vi "UHR-Fleezers Control (host) - 12.0_test_fpga_connection.vi"() -> ()   [LabVIEW 2014] (continued)
                tunnel: w2776 -> [w2807]
                tunnel: w2785 -> [w2832]
                tunnel: w2786 -> [w2833]
                tunnel: w2780 -> [w2834]
                tunnel: w2777 -> [w2831]
                tunnel: [w2893] -> w2774
                frame #0 {
                  n1965 = local read "Trap Pos. FB ON"() -> (w2789:bool)
                  n1966 = Compound Arithmetic op=AND("Flow ON\nduring dip?", "FB OFF when \nflow ON", w2789) -> (w2790:bool)
                  n1967 = case shown="True" "Move trap \nbefore dip move?" {
                    frame False {
                    }
                    frame True {
                      n1968 = property on="Trap D (MHz)" class="DigNum (strict)"("Val(Sgnl)"="Dipping D (MHz)") -> ()  [unwired: 2 in, 2 out]
                    }
                  }
                  n1969 = property on="Green ON/Interlacing" class="Bool (strict)"("Val(Sgnl)"="Green ON\nbefore dip?") -> ()  [unwired: 2 in, 2 out]
                  n1970 = property on="Sample Channel\nFlow" class="Bool (strict)"("Val(Sgnl)"="Flow ON\nduring dip?") -> ()  [unwired: 2 in, 2 out]
                  n1971 = case shown="True" w2790 {
                    frame False {
                    }
                    frame True {
                      n1972 = property on="Trap Pos. FB ON" class="Bool (strict)"("Val(Sgnl)"=FALSE ("Value (Signaling)")) -> ()  [unwired: 2 in, 2 out]
                    }
                  }
                }
                frame #1 {
                  n1973 = local read "Saved Stage Positions"() -> (w2806:dbl[][])
                  n1974 = local write "Cancel dwell"(FALSE ("Cancel dwell")) -> ()
                  n1975 = call "move to saved stage position.vi"("error in"=w2804, "Stage VISA resource name in"=w2803, "Position"="Dip Stage \nPosition", "Saved Stage Positions"=w2806) -> ("VISA resource name out"=w2801:refnum<visa-resource-name>, "error out"=w2802:errorcluster)
                }
                frame #2 {
                  n1976 = node-c288() -> (w2810:T26)  [unwired: 4 in]
                  n1977 = timed-loop {
                    timing: w2810 -> [_]
                    timing-out: [_] -> w2809
                    tunnel: [w2816] -> w2808
                    i -> [w2813]
                    stop <- w2817 stop-if-true
                    n1978 = node-c288() -> ()  [unwired: 1 in, 1 out]
                    n1979 = Greater Or Equal?(x=w2813, y="Dip Duration (s)") -> (x >= y?=w2825:bool)
                    n1980 = local read "Dip for Protein"() -> (w2818:bool)
                    n1981 = local read "Dump Beads"() -> (w2815:bool)
                    n1982 = local read "Cancel dwell"() -> (w2824:bool)
                    n1983 = local read "Pause dwell"() -> (w2821:bool)
                    n1984 = Not(x=w2818) -> (.not. x?=w2823:bool)
                    n1985 = Compound Arithmetic op=OR(w2824, w2825, w2823) -> (w2822:bool)
                    n1986 = Select(t=FALSE, s=w2821, f=w2822) -> (s? t:f=w2819:bool)
                    n1987 = Not(x=w2815) -> (.not. x?=w2814:bool)
                    n1988 = node-c288() -> ()  [unwired: 1 in, 1 out]
                    n1989 = And(x=w2818, y=w2814) -> (x .and. y?=w2816:bool)
                    n1990 = Or(x=w2819, y=w2815) -> (x .or. y?=w2817:bool)
                    "Dip Time (s)" <- w2813
                  }
                  n1991 = node-c288(w2809) -> ()  [unwired: 1 out]
                }
                frame #3 {
                  n1992 = case shown="True" w2834 {
                    tunnel: w2833 -> [_ w2839]
                    tunnel: w2832 -> [_ w2838]
                    tunnel: w2831 -> [_ w2835]
                    frame False {
                    }
                    frame True {
                      n1993 = flat-sequence {
                        tunnel: w2838 -> [w2843]
                        tunnel: w2839 -> [w2844]
                        tunnel: [w2844] -> w2837
                        tunnel: [w2843] -> w2836
                        tunnel: w2835 -> [w2840]
                        tunnel: w2837 -> [w2854]
                        tunnel: w2836 -> [w2853]
                        tunnel: w2835 -> [w2862]
                        frame #0 {
                          n1994 = local read "Sample Channel\nFlow"() -> (w2842:bool)
                          n1995 = case shown="True" w2842 {
                            tunnel: "Flow ON \nduring return\nfrom dip?" -> [w2845 w2848]
                            tunnel: w2840 -> [_ w2847]
                            frame False {
                              n1996 = case shown="True" w2845 {
                                frame False {
                                }
                                frame True {
                                n1997 = property on="Sample Channel\nFlow" class="Bool (strict)"("Val(Sgnl)"=TRUE ("Value (Signaling)")) -> ()  [unwired: 2 in, 2 out]
                                }
                              }
                            }
                            frame True {
                              n1998 = case shown="False" w2848 {
                                tunnel: w2847 -> [w2849 _]
                                frame False {
                                n1999 = property on="Trap Pos. FB ON" class="Bool (strict)"("Val(Sgnl)"=w2849) -> ()  [unwired: 2 in, 2 out]
                                n2000 = property on="Sample Channel\nFlow" class="Bool (strict)"("Val(Sgnl)"=FALSE ("Value (Signaling)")) -> ()  [unwired: 2 in, 2 out]
                                }
                                frame True {
                                }
                              }
                            }
                          }
                        }
                        frame #1 {
                          # "For turning on green laser before stage reaches lower spot"
                          n2001 = case shown="True" "Green ON\nafter start\nreturn?" {
                            frame False {
                            }
                            frame True {
                              n2002 = flat-sequence {
                                frame #0 {
                                n2003 = Multiply(x="Green delay after \nstart return (s)", y=1000.0) -> (x*y=w2859:dbl)
                                n2004 = Wait (ms)(milliseconds to wait=w2859) -> ()  [unwired: 1 out]
                                }
                                frame #1 {
                                n2005 = property on="Green ON/Interlacing" class="Bool (strict)"("Val(Sgnl)"=TRUE ("Value (Signaling)")) -> ()  [unwired: 2 in, 2 out]
                                }
                              }
                            }
                          }
                          n2006 = local read "Saved Stage Positions"() -> (w2857:dbl[][])
                          n2007 = local write "Cancel dwell"(FALSE ("Cancel dwell")) -> ()
                          n2008 = call "move to saved stage position.vi"("error in"=w2853, "Stage VISA resource name in"=w2854, "Position"="Return Stage \nPosition", "Saved Stage Positions"=w2857) -> ("error out"=w2855:errorcluster)  [unwired: 1 out]
                          n2009 = local write "Stage Control Serial Error"(w2855) -> ()
                        }
                        frame #2 {
                          n2010 = property on="Trap Pos. FB ON" class="Bool (strict)"("Val(Sgnl)"=w2862) -> ()  [unwired: 2 in, 2 out]
                          n2011 = case shown="True" "Green ON \nafter return?" {
                            frame False {
                            }
                            frame True {
                              n2012 = property on="Green ON/Interlacing" class="Bool (strict)"("Val(Sgnl)"=TRUE ("Value (Signaling)")) -> ()  [unwired: 2 in, 2 out]
                            }
                          }
                          n2013 = case shown="True" "Move trap after return?" {
                            frame False {
                            }
                            frame True {
                              n2014 = property on="Trap D (MHz)" class="DigNum (strict)"("Val(Sgnl)"="Dip Trap D 2 (MHz)") -> ()  [unwired: 2 in, 2 out]
                            }
                          }
                          n2015 = case shown="True" "Save data after return?" {
                            frame False {
                            }
                            frame True {
                              n2016 = property on="Start Saving" class="Bool (strict)"("Val(Sgnl)"=TRUE ("Value (Signaling)")) -> ()  [unwired: 2 in, 2 out]
                            }
                          }
                          n2017 = property on="Sample Channel\nFlow" class="Bool (strict)"("Val(Sgnl)"="Flow ON\nduring daq?") -> ()  [unwired: 2 in, 2 out]
                        }
                        frame #3 {
                          n2018 = node-c288() -> (w2871:T26)  [unwired: 4 in]
                          n2019 = timed-loop {
                            timing: w2871 -> [_]
                            timing-out: [_] -> w2870
                            i -> [w2872]
                            stop <- w2874 stop-if-true
                            n2020 = node-c288() -> ()  [unwired: 1 in, 1 out]
                            n2021 = local read "Dump Beads"() -> (w2873:bool)
                            n2022 = Greater Or Equal?(x=w2872, y="Dwell Duration (s)") -> (x >= y?=w2879:bool)
                            n2023 = local read "Dip for Protein"() -> (w2876:bool)
                            n2024 = Not(x=w2876) -> (.not. x?=w2875:bool)
                            n2025 = Compound Arithmetic op=OR(w2879, "Cancel dwell", w2875) -> (w2878:bool)
                            n2026 = node-c288() -> ()  [unwired: 1 in, 1 out]
                            n2027 = Select(t=FALSE, s="Pause dwell", f=w2878) -> (s? t:f=w2881:bool)
                            n2028 = Or(x=w2881, y=w2873) -> (x .or. y?=w2874:bool)
                            "Dwell Time (s)" <- w2872
                          }
                          n2029 = node-c288(w2870) -> ()  [unwired: 1 out]
                        }
                      }
                    }
                  }
                }
                frame #4 {
                  n2030 = local read "Dip for Protein"() -> (w2890:bool)
                  n2031 = local read "Tether"() -> (w2889:bool)
                  n2032 = local read "Dump Beads"() -> (w2891:bool)
                  n2033 = local write "Cancel dwell"(FALSE ("Cancel dwell")) -> ()
                  n2034 = Not(x=w2889) -> (.not. x?=w2888:bool)
                  n2035 = Not(x=w2890) -> (.not. x?=w2894:bool)
                  n2036 = Not(x="Cont. Repeat Dipping?") -> (.not. x?=w2896:bool)
                  n2037 = Compound Arithmetic op=OR(w2888, w2894, w2896, w2891) -> (w2893:bool)
                }
              }
            }
          }
        }
      }
      event "Profile": Value Change {
        n2038 = event-data() -> ()  [unwired: 1 in, 5 out]
        n2039 = flat-sequence {
          tunnel: w2905 -> [w2908]
          tunnel: w2904 -> [w2916]
          tunnel: [w2910] -> w2903
          tunnel: [w2909] -> w2902
          tunnel: [w2907] -> w2900
          tunnel: [w2906] -> w2897
          tunnel: w2903 -> [w2923]
          tunnel: w2902 -> [w2922]
          tunnel: [w2920] -> w2901
          tunnel: w2900 -> [w2921]
          tunnel: [w2919] -> w2899
          tunnel: [w2918] -> w2898
          tunnel: w2897 -> [w2918]
          tunnel: w2901 -> [w2927]
          tunnel: w2899 -> [w2926]
          tunnel: w2898 -> [w2925]
          frame #0 {
            n2040 = call "Read Stage Position.vi"("error in"=w2916, "VISA resource name in"=w2908) -> ("Current Position"=w2906:cluster{dbl, dbl, dbl}, "error out"=w2909:errorcluster, "VISA resource name out"=w2907:refnum<visa-resource-name>)  [unwired: 1 out]
            "Current Position" <- w2906
            n2041 = local write "Stage Control Serial Error"(w2909) -> ()
            n2042 = Unbundle(w2906) -> (w2913:dbl, w2915:dbl, w2911:dbl)
            n2043 = Add(x=w2915, y="Y change (mm)") -> (x+y=w2912:dbl)
            n2044 = Bundle(w2913, w2912, w2911) -> (w2910:cluster{dbl, dbl, dbl})  [unwired: 1 in]
          }
          frame #1 {
            # "move to new position and start saving"
            n2045 = local write "Stage Moving"(TRUE ("Stage Moving")) -> ()
            n2046 = local write "Start Saving"(TRUE ("Start Saving")) -> ()
            n2047 = call "Set Stage Position.vi"("Position"=w2923, "error in"=w2922, "VISA resource name in"=w2921) -> ("error out"=w2919:errorcluster, "VISA resource name out"=w2920:refnum<visa-resource-name>)  [unwired: 1 out]
          }
          frame #2 {
            # "go back to start"
            n2048 = call "Set Stage Position.vi"("Position"=w2925, "error in"=w2926, "VISA resource name in"=w2927) -> ()  [unwired: 3 out]
          }
          frame #3 {
            # "stop saving"
            n2049 = local write "Stop Saving"(TRUE ("Stop Saving")) -> ()
            n2050 = local write "Stage Moving"(FALSE ("Stage Moving")) -> ()
          }
        }
      }
      event "Move to Position 1", "Move to Position 2", "Move to Position 3", "Move to Position 4", "Move to Position 5", "Lower Ch. Cap.": Value Change {
        n2051 = event-data() -> ()  [unwired: 1 in, 5 out]
        n2052 = Or(x="Move to Position 5", y="Lower Ch. Cap.") -> (x .or. y?=w2933:bool)
        n2053 = Build Array("Move to Position 1", "Move to Position 2", "Move to Position 3", "Move to Position 4", w2933) -> (w2936:bool[])
        n2054 = Boolean Array To Number(Boolean array=w2936) -> (number=w2935:u32)
        n2055 = Logarithm Base 2(1:w2935) -> (0:w2934:dbl)
        n2056 = flat-sequence {
          tunnel: w2934 -> [w2945]
          tunnel: w2931 -> [w2943]
          tunnel: w2930 -> [w2942]
          frame #0 {
            n2057 = local read "Saved Stage Positions"() -> (w2953:dbl[][])
            n2058 = Array Subset(array=w2953, index (row)=w2945, length (row)=1 ("length"), index (col)=1 ("index"), length (col)=3 ("length")) -> (w2950:dbl[][])
            n2059 = Reshape Array(w2950, 3 ("dimension size")) -> (w2948:dbl[])
            n2060 = Array To Cluster(array=w2948) -> (cluster=w2947:cluster{"[0]":dbl, "[1]":dbl, "[2]":dbl})
            n2061 = call "Set Stage Position.vi"("Position"=w2947, "error in"=w2942, "VISA resource name in"=w2943) -> ("error out"=w2946:errorcluster)  [unwired: 2 out]
            n2062 = local write "Stage Moving"(TRUE ("Stage Moving")) -> ()
            n2063 = local write "Stage Control Serial Error"(w2946) -> ()
          }
          frame #1 {
            n2064 = local write "Stage Moving"(FALSE ("Stage Moving")) -> ()
            n2065 = call <vilib>:"Beep.vi"() -> ()  [unwired: 3 in, 9 out]
          }
        }
      }
      event "Set Current\nPos to 0,0,0": Value Change {
        # "DH is \"Define Home\""
        n2066 = event-data() -> ()  [unwired: 1 in, 6 out]
        n2067 = local write "Set Current\nPos to 0,0,0"(FALSE ("Set Current\nPos to 0,0,0")) -> ()
        n2068 = Concatenate Strings("1DH" ("string"), ";" ("string"), "2DH" ("string"), ";" ("string"), "3DH" ("string"), "\r") -> (w2961:string)
        n2069 = call-poly "VISA Configure Serial Port"("VISA resource name"=w2966, "baud rate (9600)"=u32 19200, "error in (no error)"=w2965) -> ("VISA resource name out"=w2963:refnum<visa-resource-name>, "error out"=w2962:errorcluster)  [unwired: 11 in]
        n2070 = VISA Write(VISA resource name=w2963, write buffer=w2961, error in (no error)=w2962) -> (error out=w2956:errorcluster)  [unwired: 2 out]
        n2071 = local write "Stage Control Serial Error"(w2956) -> ()
      }
      event "Got ADig bead": Value Change {
        n2072 = event-data() -> ()  [unwired: 1 in, 5 out]
        n2073 = flat-sequence {
          frame #0 {
            n2074 = local read "Cap 1 Samp Flow ON"() -> (w2972:bool)
            n2075 = case shown="True" w2972 {
              frame False {
              }
              frame True {
                n2076 = property on="Sample Channel\nFlow" class="Bool (strict)"("Val(Sgnl)"=TRUE ("Value (Signaling)")) -> ()  [unwired: 2 in, 2 out]
              }
            }
            n2077 = local write "Got ADig bead"(FALSE) -> ()
          }
          frame #1 {
            n2078 = property on="Inject Pump 3" class="Bool (strict)"("Val(Sgnl)"=FALSE ("Value (Signaling)")) -> ()  [unwired: 2 in, 2 out]
            n2079 = local write "Target"(FALSE ("Target")) -> ()
          }
          frame #2 {
            n2080 = property on="Move Cap. 1 (DNA Bottom)" class="Bool (strict)"("Val(Sgnl)"=TRUE ("Value (Signaling)")) -> ()  [unwired: 2 in, 2 out]
          }
        }
      }
      event "Force FB Script": Value Change {
        n2081 = event-data() -> ()  [unwired: 1 in, 5 out]
        n2082 = local write "Force FB Script"(FALSE ("Force FB Data\nScript")) -> ()
        n2083 = flat-sequence {
          tunnel: w2983 -> [w2987]
          tunnel: w2984 -> [w2988]
          tunnel: [w2988] -> w2979
          tunnel: [w2987] -> w2978
          tunnel: w2979 -> [w2991]
          tunnel: w2978 -> [w2990]
          tunnel: ["Trap Trig Fl."] -> w2980
          tunnel: [w3033] -> w2981
          tunnel: w2980 -> [w3033]
          tunnel: [w3037] -> w2982
          tunnel: w2981 -> [w3037]
          tunnel: w2982 -> [w3039]
          frame #0 {
            n2084 = property on="Trap D (MHz)" class="DigNum (strict)"("Val(Sgnl)"="Trap D Before Moving") -> ()  [unwired: 2 in, 2 out]
          }
          frame #1 {
            n2085 = local read "Saved Stage Positions"() -> (w2993:dbl[][])
            n2086 = local write "FB Trap Pos Offset"(0.0 ("FB Trap Pos Offset")) -> ()
            n2087 = property on="Trap Pos. FB Offset Factor" class="DigNum (strict)"("Val(Sgnl)"=i64 0 ("Value (Signaling)")) -> ()  [unwired: 2 in, 2 out]
            n2088 = local write "Stage Moving"(TRUE ("Stage Moving")) -> ()
            n2089 = call "move to saved stage position.vi"("error in"=w2990, "Stage VISA resource name in"=w2991, "Position"="Stage Position To Establish FB", "Saved Stage Positions"=w2993) -> ("error out"=w2989:errorcluster)  [unwired: 1 out]
            n2090 = local write "Stage Control Serial Error"(w2989) -> ()
          }
          frame #2 {
            n2091 = call <vilib>:"Beep.vi"("duration (msec)"=u32 100, "frequency (Hz)"=u32 20) -> ()  [unwired: 1 in, 9 out]
            n2092 = local write "Stage Moving"(FALSE ("Stage Moving")) -> ()
            n2093 = property on="Tab Control 2" class="TabCtl (strict)"("Val(Sgnl)"=T6."Feedback on Trap Position" ("Value (Signaling)")) -> ()  [unwired: 2 in, 2 out]
            n2094 = stacked-sequence {
              frame #0 {
                n2095 = Multiply(x="Wait (s)", y=u32 1000 ("milliseconds to wait")) -> (x*y=w3002:u32)
                n2096 = property on="Trap D (MHz)" class="DigNum (strict)"("Val(Sgnl)"="Starting Trap D (MHz)") -> ()  [unwired: 2 in, 2 out]
                n2097 = Wait (ms)(milliseconds to wait=w3002) -> ()  [unwired: 1 out]
              }
              frame #1 {
                n2098 = property on="Set Reading to\nSetpoint" class="Bool (strict)"("Val(Sgnl)"=TRUE ("Value (Signaling)")) -> ()  [unwired: 2 in, 2 out]
              }
            }
            n2099 = property on="Tab Control" class="TabCtl (strict)"("Val(Sgnl)"=T34."Trap Control (RF)" ("Value (Signaling)")) -> ()  [unwired: 2 in, 2 out]
          }
          frame #3 {
            n2100 = Wait (ms)(milliseconds to wait=u32 500) -> ()  [unwired: 1 out]
          }
          frame #4 {
            n2101 = property on="Trap Pos. FB ON" class="Bool (strict)"("Val(Sgnl)"=TRUE ("Value (Signaling)")) -> ()  [unwired: 2 in, 2 out]
            n2102 = Wait (ms)(milliseconds to wait=u32 250) -> ()  [unwired: 1 out]
          }
          frame #5 {
            n2103 = case shown="\"1\"" "Remove Action Offset Dropdown" {
              tunnel: TRUE ("Value (Signaling)") -> [w3014 w3022 w3030]
              frame "1" {
                n2104 = flat-sequence {
                  tunnel: w3014 -> [w3021]
                  frame #0 {
                    n2105 = local read "factor"() -> (w3016:dbl)
                    n2106 = Greater Than 0?(x=w3016) -> (x > 0?=w3020:bool)
                    n2107 = Select(t=1.0, s=w3020, f=-1.0) -> (s? t:f=w3017:dbl)
                    n2108 = Multiply(x=w3017, y=w3016) -> (x*y=w3015:dbl)
                    n2109 = local write "factor"(w3015) -> ()
                  }
                  frame #1 {
                    n2110 = property on="Remove Offset to factor" class="Bool (strict)"("Val(Sgnl)"=w3021) -> ()  [unwired: 2 in, 2 out]
                  }
                }
              }
              frame "2" {
                n2111 = flat-sequence {
                  tunnel: w3022 -> [w3029]
                  frame #0 {
                    n2112 = local read "factor"() -> (w3023:dbl)
                    n2113 = Greater Than 0?(x=w3023) -> (x > 0?=w3028:bool)
                    n2114 = Select(t=-1.0, s=w3028, f=1.0) -> (s? t:f=w3026:dbl)
                    n2115 = Multiply(x=w3023, y=w3026) -> (x*y=w3025:dbl)
                    n2116 = local write "factor"(w3025) -> ()
                  }
                  frame #1 {
                    n2117 = property on="Remove Offset to factor" class="Bool (strict)"("Val(Sgnl)"=w3029) -> ()  [unwired: 2 in, 2 out]
                  }
                }
              }
              frame "0", Default {
                n2118 = property on="Remove Action Offset" class="Bool (strict)"("Val(Sgnl)"=w3030) -> ()  [unwired: 2 in, 2 out]
              }
            }
            n2119 = case shown="False" "Trap Trig Fl." {
              frame False {
                n2120 = case shown="True" "Green ON after FB ON?" {
                  selector: "Green ON after FB ON?" -> [_ w3032]
                  frame False {
                  }
                  frame True {
                    n2121 = property on="Green ON/Interlacing" class="Bool (strict)"("Val(Sgnl)"=w3032) -> ()  [unwired: 2 in, 2 out]
                  }
                }
              }
              frame True {
              }
            }
            n2122 = Wait (ms)(milliseconds to wait=u32 250) -> ()  [unwired: 1 out]
          }
          frame #6 {
            n2123 = property on="Start Saving" class="Bool (strict)"("Val(Sgnl)"=TRUE ("Value (Signaling)")) -> ()  [unwired: 2 in, 2 out]
            n2124 = Wait (ms)(milliseconds to wait=u32 5000) -> ()  [unwired: 1 out]
          }
          frame #7 {
            w3036 = TRUE ("Value (Signaling)")
            n2125 = property on="Rem fb disp offset" class="Bool (strict)"("Val(Sgnl)"=w3036) -> ()  [unwired: 2 in, 2 out]
            n2126 = property on="Remove Offset" class="Bool (strict)"("Val(Sgnl)"=w3036) -> ()  [unwired: 2 in, 2 out]
            n2127 = Wait (ms)(milliseconds to wait=u32 100) -> ()  [unwired: 1 out]
          }
          frame #8 {
            n2128 = case shown="True" w3039 {
              frame False {
              }
              frame True {
                n2129 = local write "Trap Trig. Fl."(TRUE ("Value (Signaling)")) -> ()
              }
            }
          }
          frame #9 {
            n2130 = local read "Tether"() -> (w3042:bool)
            n2131 = And(x="Start dipping after?", y=w3042) -> (x .and. y?=w3041:bool)
            n2132 = case shown="True" w3041 {
              frame False {
              }
              frame True {
                n2133 = flat-sequence {
                  frame #0 {
                    n2134 = Multiply(x="Delay before dipping (s)", y=1000.0) -> (x*y=w3045:dbl)
                    n2135 = Wait (ms)(milliseconds to wait=w3045) -> ()  [unwired: 1 out]
                  }
                  frame #1 {
                    n2136 = property on="Dip for Protein" class="Bool (strict)"("Val(Sgnl)"=TRUE ("Value (Signaling)")) -> ()  [unwired: 2 in, 2 out]
                    n2137 = local write "Scripts"(T35."Dipping") -> ()
                  }
                }
              }
            }
          }
        }
      }
      event "Rupture Script": Value Change {
        n2138 = event-data() -> ()  [unwired: 1 in, 5 out]
        n2139 = local write "Rupture Script"(FALSE ("Rupture Script")) -> ()
        n2140 = flat-sequence {
          frame #0 {
            w3051 = TRUE
            w3056 = FALSE
            # "Number 6 for now is the\nrupture-experiment\nparameters."
            n2141 = local read "Starting Trap D (MHz)"() -> (w3057:dbl)
            n2142 = local write "Restart DMA? (AOD)"(w3056) -> ()
            n2143 = Replace Array Subset(array=u32[] [0] ("Index Values"), new element=6, index=0) -> (w3052:u32[])
            n2144 = local write "Save scans"(w3056) -> ()
            n2145 = property on="Trap D (MHz)" class="DigNum (strict)"("Val(Sgnl)"=w3057) -> ()  [unwired: 2 in, 2 out]
            n2146 = property on="Saved AOD Raster Scan Parameter Sets" class="Arr (strict)"("Index Values"=w3052) -> ()  [unwired: 2 in, 2 out]
            n2147 = property on="Start Saving" class="Bool (strict)"("Val(Sgnl)"=w3051) -> ()  [unwired: 2 in, 2 out]
            n2148 = property on="Green ON/Interlacing" class="Bool (strict)"("Val(Sgnl)"=w3051) -> ()  [unwired: 2 in, 2 out]
          }
          frame #1 {
            n2149 = property on="Load parameters" class="Bool (strict)"("Val(Sgnl)"=TRUE ("Value (Signaling)")) -> ()  [unwired: 2 in, 2 out]
          }
        }
      }
      event "Fixed Traps Script": Value Change {
        n2150 = event-data() -> ()  [unwired: 1 in, 5 out]
        n2151 = local write "Fixed Traps Script"(FALSE ("Fixed Traps Data\nScript")) -> ()
        n2152 = flat-sequence {
          frame #0 {
            n2153 = case shown="True" "Green ON" {
              frame False {
              }
              frame True {
                n2154 = property on="Green ON/Interlacing" class="Bool (strict)"("Val(Sgnl)"=TRUE) -> ()  [unwired: 2 in, 2 out]
              }
            }
            n2155 = local write "Offset (nm)"(0.0 ("Offset (nm)")) -> ()
            n2156 = property on="Sample Channel\nFlow" class="Bool (strict)"("Val(Sgnl)"=FALSE ("Value (Signaling)")) -> ()  [unwired: 2 in, 2 out]
            n2157 = property on="Trap D (MHz)" class="DigNum (strict)"("Val(Sgnl)"="Fixed Traps Trap Delta (MHz)") -> ()  [unwired: 2 in, 2 out]
          }
          frame #1 {
            n2158 = Wait (ms)(milliseconds to wait=u32 1000) -> ()  [unwired: 1 out]
          }
          frame #2 {
            n2159 = local write "Start Saving"(TRUE ("Start Saving")) -> ()
          }
          frame #3 {
            n2160 = local read "Bead Sep. Int. Time (s)"() -> (w3067:dbl)
            n2161 = Multiply(x=w3067, y=1000.0) -> (x*y=w3069:dbl)
            n2162 = Wait (ms)(milliseconds to wait=w3069) -> ()  [unwired: 1 out]
          }
          frame #4 {
            n2163 = property on="Remove Offset" class="Bool (strict)"("Val(Sgnl)"=TRUE ("Value (Signaling)")) -> ()  [unwired: 2 in, 2 out]
          }
          frame #5 {
            n2164 = property on="Dip for Protein" class="Bool (strict)"("Val(Sgnl)"="Start dipping after?") -> ()  [unwired: 2 in, 2 out]
          }
        }
      }
      event "Got DNA bead": Value Change {
        n2165 = event-data() -> ()  [unwired: 1 in, 5 out]
        n2166 = flat-sequence {
          frame #0 {
            w3073 = FALSE ("Key Focus")
            n2167 = local read "Daq spot flow on"() -> (w3074:bool)
            n2168 = case shown="True" w3074 {
              frame False {
              }
              frame True {
                n2169 = property on="Sample Channel\nFlow" class="Bool (strict)"("Val(Sgnl)"=TRUE ("Value (Signaling)")) -> ()  [unwired: 2 in, 2 out]
              }
            }
            n2170 = local write "Got DNA bead"(w3073) -> ()
            n2171 = property on="Got DNA bead" class="Bool (strict)"("Key Focus"=w3073) -> ()  [unwired: 2 in, 2 out]
          }
          frame #1 {
            n2172 = property on="Inject Pump 1" class="Bool (strict)"("Val(Sgnl)"=FALSE ("Value (Signaling)")) -> ()  [unwired: 2 in, 2 out]
          }
          frame #2 {
            n2173 = property on="Cal/Data Acq. Spot" class="Bool (strict)"("Val(Sgnl)"=TRUE ("Value (Signaling)")) -> ()  [unwired: 2 in, 2 out]
          }
        }
      }
      event "Take Stepping Data": Value Change {
        n2174 = event-data() -> ()  [unwired: 1 in, 5 out]
        n2175 = local read "Save ave N"() -> (w3086:dbl)
        n2176 = flat-sequence {
          tunnel: w3086 -> [w3088]
          tunnel: [w3088] -> w3081
          tunnel: [w3090] -> w3082
          tunnel: w3081 -> [w3090]
          tunnel: [w3092] -> w3083
          tunnel: w3082 -> [w3092]
          tunnel: [w3095] -> w3084
          tunnel: w3083 -> [w3095]
          tunnel: [w3097] -> w3085
          tunnel: w3084 -> [w3097]
          tunnel: [w3099] -> w3079
          tunnel: w3085 -> [w3099]
          tunnel: w3079 -> [w3102]
          tunnel: [w3102] -> w3078
          tunnel: w3078 -> [w3103]
          tunnel: [w3103] -> w3080
          tunnel: w3080 -> [w3109]
          frame #0 {
            n2177 = property on="Save ave N" class="DigNum (strict)"("Val(Sgnl)"="Save ave factor") -> ()  [unwired: 2 in, 2 out]
          }
          frame #1 {
            n2178 = Wait (ms)(milliseconds to wait=u32 100) -> ()  [unwired: 1 out]
          }
          frame #2 {
            n2179 = local read "Offset 2 Start (MHz)"() -> (w3094:dbl)
            n2180 = property on="Saved AOD Raster Scan Parameter Sets" class="Arr (strict)"("Index Values"=u32[] [2]) -> ()  [unwired: 2 in, 2 out]
            n2181 = property on="Trap D (MHz)" class="DigNum (strict)"("Val(Sgnl)"=w3094) -> ()  [unwired: 2 in, 2 out]
          }
          frame #3 {
            n2182 = property on="Load parameters" class="Bool (strict)"("Val(Sgnl)"=TRUE ("Value (Signaling)")) -> ()  [unwired: 2 in, 2 out]
          }
          frame #4 {
            n2183 = Wait (ms)(milliseconds to wait=u32 100) -> ()  [unwired: 1 out]
          }
          frame #5 {
            n2184 = property on="Trap Raster Scan" class="Bool (strict)"("Val(Sgnl)"=TRUE ("Value (Signaling)")) -> ()  [unwired: 2 in, 2 out]
          }
          frame #6 {
            n2185 = Wait (ms)(milliseconds to wait=u32 1000) -> ()  [unwired: 1 out]
          }
          frame #7 {
            n2186 = while {
              stop <- w3106 stop-if-true
              n2187 = local read "Raster Scanning..."() -> (w3108:bool)
              n2188 = local read "Saving..."() -> (w3107:bool)
              n2189 = Not(x=w3107) -> (.not. x?=w3104:bool)
              n2190 = Not(x=w3108) -> (.not. x?=w3105:bool)
              n2191 = And(x=w3105, y=w3104) -> (x .and. y?=w3106:bool)
            }
          }
          frame #8 {
            n2192 = property on="Save ave N" class="DigNum (strict)"("Val(Sgnl)"=w3109) -> ()  [unwired: 2 in, 2 out]
          }
        }
      }
      event "Step Size (nm)": Value Change {
        n2193 = event-data() -> ()  [unwired: 1 in, 5 out]
        n2194 = flat-sequence {
          frame #0 {
            n2195 = property on="Saved AOD Raster Scan Parameter Sets" class="Arr (strict)"("Index Values"=u32[] [1]) -> ()  [unwired: 2 in, 2 out]
          }
          frame #1 {
            n2196 = Multiply(x="N Steps", y="Step Size (nm)") -> (x*y=w3111:dbl)
            n2197 = property on="Scan Speed AOD (nm/s) 2" class="DigNum (strict)"("Value"="Step Size (nm)") -> ()  [unwired: 2 in, 2 out]
            n2198 = property on="Step Size AOD (nm) 2" class="DigNum (strict)"("Value"="Step Size (nm)") -> ()  [unwired: 2 in, 2 out]
            n2199 = property on="Scan Range AOD (nm) 2" class="DigNum (strict)"("Value"=w3111) -> ()  [unwired: 2 in, 2 out]
          }
        }
      }
      event "Take Detection Laser\nImage": Value Change {
        n2200 = event-data() -> ()  [unwired: 1 in, 5 out]
        n2201 = flat-sequence {
          tunnel: [w3139] -> w3129
          tunnel: [w3138] -> w3122
          tunnel: [w3137] -> w3114
          tunnel: [w3142] -> w3130
          tunnel: w3129 -> [w3142]
          tunnel: [w3141] -> w3123
          tunnel: w3122 -> [w3141]
          tunnel: [w3140] -> w3115
          tunnel: w3114 -> [w3140]
          tunnel: [w3146] -> w3131
          tunnel: w3130 -> [w3146]
          tunnel: [w3145] -> w3124
          tunnel: w3123 -> [w3145]
          tunnel: [w3144] -> w3116
          tunnel: w3115 -> [w3144]
          tunnel: [w3152] -> w3132
          tunnel: w3131 -> [w3152]
          tunnel: [w3151] -> w3125
          tunnel: w3124 -> [w3151]
          tunnel: [w3150] -> w3117
          tunnel: w3116 -> [w3150]
          tunnel: [w3156] -> w3133
          tunnel: w3132 -> [w3156]
          tunnel: [w3155] -> w3126
          tunnel: w3125 -> [w3155]
          tunnel: [w3154] -> w3118
          tunnel: w3117 -> [w3154]
          tunnel: [w3160] -> w3134
          tunnel: w3133 -> [w3160]
          tunnel: [w3159] -> w3127
          tunnel: w3126 -> [w3159]
          tunnel: [w3158] -> w3119
          tunnel: w3118 -> [w3158]
          tunnel: [w3164] -> w3135
          tunnel: w3134 -> [w3164]
          tunnel: [w3163] -> w3128
          tunnel: w3127 -> [w3163]
          tunnel: [w3162] -> w3120
          tunnel: w3119 -> [w3162]
          tunnel: w3135 -> [w3170]
          tunnel: w3128 -> [w3169]
          tunnel: [w3167] -> w3121
          tunnel: w3120 -> [w3167]
          tunnel: w3121 -> [w3171]
          frame #0 {
            n2202 = local read "Laser interlacing mode (all lasers)"() -> (w3138:enum32{"Laser ON", "Laser OFF", "Interlace"})
            n2203 = local read "Green ON/Interlacing"() -> (w3139:bool)
            n2204 = local read "Green FB On/Off"() -> (w3137:bool)
          }
          frame #1 {
            n2205 = property on="Green FB On/Off" class="Bool (strict)"("Val(Sgnl)"=FALSE ("Value (Signaling)")) -> ()  [unwired: 2 in, 2 out]
          }
          frame #2 {
            n2206 = property on="Green ON/Interlacing" class="Bool (strict)"("Val(Sgnl)"=TRUE ("Value (Signaling)")) -> ()  [unwired: 2 in, 2 out]
            n2207 = property on="Flip Green Filter" class="Bool (strict)"("Val(Sgnl)"=TRUE ("Value (Signaling)")) -> ()  [unwired: 2 in, 2 out]
            n2208 = property on="Laser interlacing mode (all lasers)" class="RadioBtnsControl (strict)"("Val(Sgnl)"=enum32{"Laser ON", "Laser OFF", "Interlace"}."Laser ON" ("Value (Signaling)")) -> ()  [unwired: 2 in, 2 out]
          }
          frame #3 {
            n2209 = Wait (ms)(milliseconds to wait=u32 500) -> ()  [unwired: 1 out]
          }
          frame #4 {
            n2210 = property on="Confocal\nImage" class="Bool (strict)"("Val(Sgnl)"=TRUE ("Value (Signaling)")) -> ()  [unwired: 2 in, 2 out]
          }
          frame #5 {
            n2211 = Wait (ms)(milliseconds to wait=u32 2000) -> ()  [unwired: 1 out]
          }
          frame #6 {
            n2212 = while {
              stop <- w3165 stop-if-true
              n2213 = local read "Saving..."() -> (w3166:bool)
              n2214 = Not(x=w3166) -> (.not. x?=w3165:bool)
            }
          }
          frame #7 {
            n2215 = property on="Flip Green Filter" class="Bool (strict)"("Val(Sgnl)"=TRUE ("Value (Signaling)")) -> ()  [unwired: 2 in, 2 out]
            n2216 = property on="Green ON/Interlacing" class="Bool (strict)"("Val(Sgnl)"=w3170) -> ()  [unwired: 2 in, 2 out]
            n2217 = property on="Laser interlacing mode (all lasers)" class="RadioBtnsControl (strict)"("Val(Sgnl)"=w3169) -> ()  [unwired: 2 in, 2 out]
          }
          frame #8 {
            n2218 = property on="Green FB On/Off" class="Bool (strict)"("Val(Sgnl)"=w3171) -> ()  [unwired: 2 in, 2 out]
          }
        }
      }
      event "Stop All": Value Change {
        n2219 = event-data() -> ()  [unwired: 1 in, 5 out]
        n2220 = local read "Stop All"() -> (w3172:bool)
      }
    }
    n2221 = node-c288() -> ()  [unwired: 1 in, 1 out]
  }
  n2222 = node-c288() -> (w139:T26)  [unwired: 4 out]
  n2223 = timed-loop "Mouse control: trap position (AOM deflection), set confocal spot from image" {
    tunnel: [w3174] -> w224
    tunnel: w51 -> [w3173]
    timing: w139 -> [_]
    timing-out: [_] -> w138
    stop <- w3174 stop-if-true
    n2224 = node-c288() -> ()  [unwired: 2 out]
    n2225 = event shown="[0] \"Pane\": Mouse Down" {
      selector: _ -> [_ _]
      dyn-events: _ -> [_ _]
      timeout: _ -> [_ _]
      tunnel: w3173 -> [w3177 _]
      event Mouse Down {
        n2226 = event-data() -> ("Time"=w3179:u32, "Coords"=w3178:T7, "Button"=w3180:u16)  [unwired: 6 out]
        n2227 = case shown="1" w3180 {
          tunnel: w3179 -> [_ _ w3319]
          tunnel: w3178 -> [_ w3185 w3317]
          tunnel: w3177 -> [_ _ w3315]
          frame 0, Default {
          }
          frame 1 {
            n2228 = property on="APD 2" class="ImageControl"() -> ("Displayed Image Position"=w3199:cluster{"Left":i32, "Top":i32})  [unwired: 2 in, 2 out]
            n2229 = control-ref of="Primary Video Display"() -> (w3192:refnum<vi>)
            n2230 = property on="APD 1" class="ImageControl"() -> ("Displayed Image Position"=w3228:cluster{"Left":i32, "Top":i32})  [unwired: 2 in, 2 out]
            n2231 = property on="Detection Laser X" class="ImageControl"() -> ("Displayed Image Position"=w3225:cluster{"Left":i32, "Top":i32})  [unwired: 2 in, 2 out]
            n2232 = property on="Detection Laser Y" class="ImageControl"() -> ("Displayed Image Position"=w3224:cluster{"Left":i32, "Top":i32})  [unwired: 2 in, 2 out]
            n2233 = property on="APD 2" class="ImageControl"() -> ("Displayed Image Size"=w3198:cluster{"Width":u32, "Height":u32})  [unwired: 2 in, 2 out]
            n2234 = property on="APD 1" class="ImageControl"() -> ("Displayed Image Size"=w3226:cluster{"Width":u32, "Height":u32})  [unwired: 2 in, 2 out]
            n2235 = property on="Detection Laser X" class="ImageControl"() -> ("Displayed Image Size"=w3227:cluster{"Width":u32, "Height":u32})  [unwired: 2 in, 2 out]
            n2236 = property on="Detection Laser Y" class="ImageControl"() -> ("Displayed Image Size"=w3223:cluster{"Width":u32, "Height":u32})  [unwired: 2 in, 2 out]
            n2237 = property class="ImageControl"(reference=w3192) -> ("Displayed Image Position"=w3190:cluster{"Left":i32, "Top":i32})  [unwired: 1 in, 2 out]
            n2238 = property class="ImageControl"(reference=w3192) -> ("Displayed Image Size"=w3191:cluster{"Width":u32, "Height":u32})  [unwired: 1 in, 2 out]
            n2239 = Unbundle By Name(w3198) -> ("Width"=w3195:u32, "Height"=w3194:u32)
            n2240 = Unbundle By Name(w3199) -> ("Left"=w3197:i32, "Top"=w3196:i32)
            n2241 = Unbundle By Name(w3226) -> ("Width"=w3220:u32, "Height"=w3219:u32)
            n2242 = Unbundle By Name(w3227) -> ("Width"=w3216:u32, "Height"=w3215:u32)
            n2243 = Unbundle By Name(w3223) -> ("Width"=w3212:u32, "Height"=w3211:u32)
            n2244 = Unbundle By Name(w3228) -> ("Left"=w3222:i32, "Top"=w3221:i32)
            n2245 = Unbundle By Name(w3225) -> ("Left"=w3218:i32, "Top"=w3217:i32)
            n2246 = Unbundle By Name(w3224) -> ("Left"=w3214:i32, "Top"=w3213:i32)
            n2247 = Bundle("Left"=w3197, "Top"=w3196, "Width"=w3195, "Height"=w3194) -> (w3193:T36)  [unwired: 1 in]
            n2248 = Bundle("Left"=w3222, "Top"=w3221, "Width"=w3220, "Height"=w3219) -> (w3210:T36)  [unwired: 1 in]
            n2249 = Bundle("Left"=w3218, "Top"=w3217, "Width"=w3216, "Height"=w3215) -> (w3209:T36)  [unwired: 1 in]
            n2250 = Bundle("Left"=w3214, "Top"=w3213, "Width"=w3212, "Height"=w3211) -> (w3208:T36)  [unwired: 1 in]
            n2251 = Unbundle By Name(w3191) -> ("Width"=w3187:u32, "Height"=w3186:u32)
            n2252 = Unbundle By Name(w3190) -> ("Left"=w3189:i32, "Top"=w3188:i32)
            n2253 = Build Cluster Array(w3193, w3210, w3209, w3208) -> (w3207:T37)
            n2254 = Bundle("Left"=w3189, "Top"=w3188, "Width"=w3187, "Height"=w3186) -> (w3182:T36)  [unwired: 1 in]
            n2255 = for {
              tunnel: w3185 -> [w3261]
              tunnel: w3207 -> [w3262] mode=indexing
              shift-right: [w3259] -> w3205
              shift-left: TRUE -> [w3260]
              shift-right: [w3258] -> w3203
              shift-left: _ -> [w3254]
              shift-right: [w3257] -> w3202
              shift-left: _ -> [w3253]
              shift-right: [w3256] -> w3201
              shift-left: _ -> [w3252]
              shift-right: [w3255] -> w3200
              shift-left: _ -> [w3251]
              n2256 = case shown="True" w3260 {
                selector: w3260 -> [w3267 _]
                tunnel: w3262 -> [_ w3276]
                tunnel: w3261 -> [_ w3274]
                tunnel: [w3267 w3272] -> w3259
                tunnel: [w3266 w3271] -> w3258
                tunnel: [w3265 w3270] -> w3257
                tunnel: [w3264 w3269] -> w3256
                tunnel: [w3263 w3268] -> w3255
                tunnel: w3254 -> [w3266 _]
                tunnel: w3253 -> [w3265 _]
                tunnel: w3252 -> [w3264 _]
                tunnel: w3251 -> [w3263 _]
                frame False {
                }
                frame True {
                  n2257 = Unbundle(w3276) -> (w3275:T36)
                  n2258 = call "isclickinwindow.vi"("Image Param"=w3275, "Point32"=w3274) -> ("4 Y"=w3268:i32, "3 Height"=w3269:i32, "2 X"=w3270:i32, "1 Width"=w3271:i32, "In image?"=w3273:bool)  [unwired: 1 in]
                  n2259 = Not(x=w3273) -> (.not. x?=w3272:bool)
                }
              }
            }
            n2260 = call "isclickinwindow.vi"("Image Param"=w3182, "Point32"=w3185) -> ("4 Y"=w3183:i32, "2 X"=w3184:i32, "In image?"=w3181:bool)  [unwired: 1 in, 2 out]
            n2261 = case shown="True" w3181 {
              tunnel: w3184 -> [_ w3232]
              tunnel: w3183 -> [_ w3235]
              frame False {
              }
              frame True {
                w3244 = 2
                n2262 = Subtract(x=480, y=w3235) -> (x-y=w3234:i32)
                n2263 = Unbundle("Target size") -> ("Width"=w3245:dbl, "Height"=w3243:dbl)
                n2264 = Subtract(x=w3232, y=2) -> (x-y=w3231:i32)
                n2265 = Divide(x=w3243, y=w3244) -> (x/y=w3241:dbl)
                n2266 = Divide(x=w3245, y=w3244) -> (x/y=w3242:dbl)
                n2267 = Subtract(x=w3231, y=w3242) -> (x-y=w3240:dbl)
                n2268 = Add(x=w3231, y=w3242) -> (x+y=w3238:dbl)
                n2269 = Subtract(x=w3234, y=w3241) -> (x-y=w3239:dbl)
                n2270 = Add(x=w3234, y=w3241) -> (x+y=w3237:dbl)
                n2271 = Bundle(w3231, w3234) -> (w3247:cluster{i32, i32})  [unwired: 1 in]
                n2272 = Bundle(w3240, w3239, w3238, w3237) -> (w3229:cluster{dbl, dbl, dbl, dbl})  [unwired: 1 in]
                n2273 = case shown="True" "Set target" {
                  tunnel: w3247 -> [_ w3250]
                  tunnel: w3229 -> [_ w3248]
                  frame False {
                  }
                  frame True {
                    n2274 = local write "Target coordinates"(w3248) -> ()
                    n2275 = local write "Set target"(FALSE ("Set target")) -> ()
                    "Video coordinates" <- w3250
                  }
                }
              }
            }
            n2276 = Not(x=w3205) -> (.not. x?=w3204:bool)
            n2277 = case shown="True" w3204 {
              tunnel: w3202 -> [_ w3290]
              tunnel: w3200 -> [_ w3289]
              tunnel: w3203 -> [_ w3288]
              tunnel: w3201 -> [_ w3287]
              frame False {
              }
              frame True {
                w3277 = FALSE ("Get Point")
                n2278 = local read "Scan lines (y)"() -> (w3292:u64)
                n2279 = disable-structure shown="Disabled" {
                  frame Disabled {
                  }
                  frame Enabled {
                  }
                }
                n2280 = local read "Actual MCL Inc (V)"() -> (w3286:dbl)
                n2281 = local read "Scan steps (MCL)"() -> (w3291:u64)
                n2282 = Divide "Y Pix/step"(x=w3287, y=w3292) -> (x/y=w3299:dbl)
                n2283 = Divide "Y V/pix"(x=w3286, y=w3299) -> (x/y=w3298:dbl)
                n2284 = Divide "Y half step offset"(x=w3286, y=2.0) -> (x/y=w3300:dbl)
                n2285 = Divide "X pix/step"(x=w3288, y=w3291) -> (x/y=w3297:dbl)
                n2286 = Negate(x=w3300) -> (-x=w3301:dbl)
                n2287 = local read "Initial Y"() -> (w3307:dbl)
                n2288 = Multiply(x=w3289, y=w3298) -> (x*y=w3308:dbl)
                n2289 = Divide "X half step offset"(x=w3286, y=2.0) -> (x/y=w3294:dbl)
                n2290 = Divide "X V/pix"(x=w3286, y=w3297) -> (x/y=w3296:dbl)
                n2291 = Multiply(x=w3286, y=w3291) -> (x*y=w3303:dbl)
                n2292 = Compound Arithmetic op=ADD(w3301, w3308, w3307) -> (w3278:dbl)
                "Pointer Y (V)" <- w3278
                n2293 = Multiply(x=w3296, y=w3290) -> (x*y=w3305:dbl)
                n2294 = Negate(x=w3294) -> (-x=w3293:dbl)
                n2295 = local read "Initial X"() -> (w3306:dbl)
                n2296 = Negate(x=w3305) -> (-x=w3304:dbl)
                n2297 = Compound Arithmetic op=ADD(w3293, w3303, w3306, w3304) -> (w3279:dbl)
                "Pointer X (V)" <- w3279
                n2298 = case shown="True" "Set High F Confocal Spot (X-Y)" {
                  tunnel: w3279 -> [_ w3309]
                  tunnel: w3278 -> [_ w3310]
                  frame False {
                  }
                  frame True {
                    "Confocal Y 2 (V)" <- w3310
                    "Confocal X 2 (V)" <- w3309
                  }
                }
                n2299 = Or(x="Set X Only", y="Set Confocal Spot (X-Y)") -> (x .or. y?=w3282:bool)
                n2300 = Or(x="Set Confocal Spot (X-Y)", y="Set Y Only") -> (x .or. y?=w3281:bool)
                n2301 = case shown="True" w3282 {
                  tunnel: w3279 -> [_ w3311]
                  frame False {
                  }
                  frame True {
                    n2302 = property on="AO2" class="Slide (strict)"("Val(Sgnl)"=w3311) -> ()  [unwired: 2 in, 2 out]
                    "Confocal X 1 (V)" <- w3311
                  }
                }
                n2303 = case shown="True" w3281 {
                  tunnel: w3278 -> [_ w3312]
                  frame False {
                  }
                  frame True {
                    n2304 = property on="AO1" class="Slide (strict)"("Val(Sgnl)"=w3312) -> ()  [unwired: 2 in, 2 out]
                    "Confocal Y 1 (V)" <- w3312
                  }
                }
                n2305 = local write "Set High F Confocal Spot (X-Y)"(w3277) -> ()
                n2306 = local write "Set Confocal Spot (X-Y)"(w3277) -> ()
                n2307 = local write "Set X Only"(w3277) -> ()
                n2308 = local write "Set Y Only"(w3277) -> ()
              }
            }
          }
          frame 3 {
            n2309 = local read "BD 2 Frequency 1 (MHz)"() -> (w3313:dbl)
            n2310 = local read "BD 1 Frequency 1 (MHz)"() -> (w3314:dbl)
            n2311 = local write "Manipulating Trap"(TRUE ("Manipulating Trap")) -> ()
            n2312 = local write "Coords"(T7 {"Horizontal"=0, "Vertical"=0} ("Coords")) -> ()
            n2313 = while {
              tunnel: w3319 -> [w3324]
              tunnel: w3317 -> [w3323]
              tunnel: w3315 -> [w3322]
              tunnel: w3314 -> [w3321]
              tunnel: w3313 -> [w3320]
              stop <- w3325 stop-if-true
              n2314 = event shown="[0] \"Pane\": Mouse Move" {
                selector: _ -> [_ _]
                dyn-events: _ -> [_ _]
                timeout: _ -> [_ _]
                tunnel: ["Force Manip Abort" w3389] -> w3325
                tunnel: w3324 -> [w3332 _]
                tunnel: w3323 -> [w3330 _]
                tunnel: w3322 -> [w3329 _]
                tunnel: w3321 -> [w3328 _]
                tunnel: w3320 -> [w3327 _]
                event Mouse Move {
                  n2315 = event-data() -> ("Time"=w3333:u32, "Coords"=w3334:T7)  [unwired: 3 out]
                  n2316 = Less?(x=w3333, y=w3332) -> (x < y?=w3331:bool)
                  n2317 = case "Makes sure old motion events prior to mouse click aren't used" shown="False" w3331 {
                    tunnel: w3334 -> [w3376 _]
                    tunnel: w3330 -> [w3377 _]
                    tunnel: w3329 -> [w3354 _]
                    tunnel: w3328 -> [w3350 _]
                    tunnel: w3327 -> [w3349 _]
                    frame False {
                      n2318 = Subtract(x=w3376, y=w3377) -> (x-y=w3375:T7)
                      "Coords" <- w3375
                      n2319 = local read "Y RF Frequency Limits (MHz)"() -> (w3335:T17)
                      n2320 = To Double Precision Float(number=w3375) -> (double precision float=w3374:cluster{"Horizontal":dbl, "Vertical":dbl})
                      n2321 = Multiply(x=cluster{"Horizontal":dbl, "Vertical":dbl} {"Horizontal"=-1.0, "Vertical"=1.0}, y="Manipulation Scaling") -> (x*y=w3370:cluster{"Horizontal":dbl, "Vertical":dbl})
                      n2322 = local read "X RF Frequency Limits (MHz)"() -> (w3336:T17)
                      n2323 = Multiply(x=w3374, y=w3370) -> (x*y=w3372:cluster{"Horizontal":dbl, "Vertical":dbl})
                      n2324 = Unbundle By Name(w3372) -> ("Horizontal"=w3367:dbl, "Vertical"=w3371:dbl)
                      n2325 = Unbundle By Name(w3335) -> ("Maximum"=w3338:dbl, "Minimum"=w3337:dbl)
                      n2326 = Boolean To (0,1)(Boolean="Manip. X?") -> (0, 1=w3365:i16)
                      n2327 = Boolean To (0,1)(Boolean="Manip. Y?") -> (0, 1=w3362:i16)
                      n2328 = local read "BD 1 Frequency 2 (MHz)"() -> (w3352:dbl)
                      n2329 = Multiply(x=w3371, y=w3362) -> (x*y=w3364:dbl)
                      n2330 = Multiply(x=w3365, y=w3367) -> (x*y=w3368:dbl)
                      n2331 = local read "BD 2 Frequency 2 (MHz)"() -> (w3351:dbl)
                      n2332 = Unbundle By Name(w3336) -> ("Maximum"=w3340:dbl, "Minimum"=w3339:dbl)
                      n2333 = Add(x=w3349, y=w3364) -> (x+y=w3342:dbl)
                      n2334 = Add(x=w3350, y=w3368) -> (x+y=w3344:dbl)
                      n2335 = In Range and Coerce(upper limit=w3340, x=w3344, lower limit=w3339) -> (coerced(x)=w3343:dbl)  [unwired: 1 out]
                      n2336 = In Range and Coerce(upper limit=w3338, x=w3342, lower limit=w3337) -> (coerced(x)=w3341:dbl)  [unwired: 1 out]
                      n2337 = Subtract(x=w3343, y=w3352) -> (x-y=w3361:dbl)
                      n2338 = Subtract(x=w3341, y=w3351) -> (x-y=w3360:dbl)
                      n2339 = Square(x=w3361) -> (x^2=w3359:dbl)
                      n2340 = Square(x=w3360) -> (x^2=w3358:dbl)
                      n2341 = Add(x=w3359, y=w3358) -> (x+y=w3357:dbl)
                      n2342 = Square Root(x=w3357) -> (sqrt(x)=w3353:dbl)
                      n2343 = In Range and Coerce(upper limit="Limit Max (MHz)", x=w3353, lower limit="Limit Min (MHz)") -> (In Range?=w3346:bool)  [unwired: 1 out]
                      n2344 = Not(x="Limits Enable") -> (.not. x?=w3345:bool)
                      n2345 = Or(x=w3346, y=w3345) -> (x .or. y?=w3347:bool)
                      n2346 = case shown="True" w3347 {
                        tunnel: w3354 -> [_ w3387]
                        tunnel: w3353 -> [_ w3378]
                        tunnel: w3343 -> [_ w3385]
                        tunnel: w3352 -> [_ w3384]
                        tunnel: w3341 -> [_ w3383]
                        tunnel: w3351 -> [_ w3382]
                        tunnel: w3336 -> [_ w3380]
                        tunnel: w3335 -> [_ w3379]
                        frame False {
                        }
                        frame True {
                          n2347 = local read "BD 1 Frequency 3 (MHz)"() -> (w3386:dbl)
                          n2348 = local read "BD 2 Frequency 3 (MHz)"() -> (w3381:dbl)
                          n2349 = local write "Trap D (MHz)"(w3378) -> ()
                          n2350 = call "set RF board frequency - interlace.vi"("Board 2 Frequency Limits"=w3379, "Board 1 Frequency Limits"=w3380, "FPGA VI Reference In"=w3387, "Board 2 Frequency 3 (MHz)"=w3381, "Board 1 Frequency 3 (MHz)"=w3386, "Board 2 Frequency 2 (MHz)"=w3382, "Board 2 Frequency 1 (MHz)"=w3383, "Board 1 Frequency 2 (MHz)"=w3384, "Board 1 Frequency 1  (MHz)"=w3385) -> ()  [unwired: 1 in, 2 out]
                          n2351 = local write "BD 2 Frequency 1 (MHz)"(w3383) -> ()
                          n2352 = local write "BD 1 Frequency 1 (MHz)"(w3385) -> ()
                        }
                      }
                    }
                    frame True {
                    }
                  }
                }
                event Mouse Up {
                  n2353 = event-data() -> ("Button"=w3388:u16)  [unwired: 8 out]
                  n2354 = case shown="3" w3388 {
                    tunnel: [FALSE TRUE] -> w3389
                    frame 0, Default {
                    }
